vi "Begin.vi"(11 "Image Size":T1=enum."160x120") -> (0 "error out":errorcluster)   [LabVIEW 2012]
doc: "Called before other user functions, this VI is expected to open initial I/O refnums, load in file data, and do all program initialization. Notice that the <B>error out</B> terminal is simply used for data flow. Wiring it to other structures or subVIs ensures that this VI runs first."
uses:
  <vilib>/Rock Robotics/WPI/Camera/WPI_CameraImageSize.ctl
  <vilib>/Rock Robotics/WPI/Camera/WPI_CameraWhite Balance Values.ctl
  <vilib>/Rock Robotics/WPI/Camera/WPI_CameraExposure Values.ctl
  <vilib>/Rock Robotics/WPI/Camera/WPI_CameraFrameRate.ctl
  <vilib>/Rock Robotics/WPI/DriverStation/WPI_DriverStationRobotMode2.ctl
  <vilib>/Rock Robotics/SystemInterfaces/DIO/FPGA_DIOChannel.ctl
  <vilib>/Rock Robotics/SystemInterfaces/AI/FPGA_AIGyroChannel.ctl
  <vilib>/Rock Robotics/WPI/Relay/WPI_RelayDirection.ctl
  <vilib>/Rock Robotics/SystemInterfaces/DIO/FPGA_DIORelayChannel.ctl
  <vilib>/Rock Robotics/SystemInterfaces/DIO/FPGA_DIOPWMChannel.ctl
  <vilib>/Rock Robotics/WPI/Joystick/WPI_JoystickDeviceEnum.ctl
  <vilib>/Rock Robotics/SystemInterfaces/Typedef/FPGA_TypedefDigitalModule.ctl
  <vilib>/Rock Robotics/SystemInterfaces/AI/FPGA_AIChannel.ctl
  Robot Global Data.vi
  <vilib>/Rock Robotics/WPI/MotorControl/WPI_MotorControlOpen Victor.vi
  <vilib>/Rock Robotics/WPI/MotorControl/WPI_MotorControlOpen Jaguar.vi
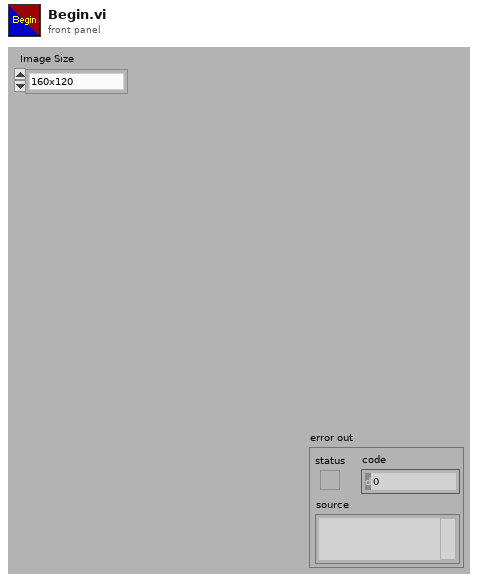
[diagram p1: front panel]
types:
  T1 = typedef "WPI_CameraImageSize.ctl" = enum16{"640x480", "320x240", "160x120"}
  T2 = typedef "FPGA_AIChannel.ctl" = enum8{"AI 1", "AI 2", "AI 3", "AI 4", "AI 5", "AI 6", "AI 7", "AI 8", "Invalid"}
  T3 = typedef "FPGA_TypedefDigitalModule.ctl" = enum16{"Digital Module 1", "Digital Module 2"}
  T4 = typedef "FPGA_DIOPWMChannel.ctl" = enum8{"PWM 1", "PWM 2", "PWM 3", "PWM 4", "PWM 5", "PWM 6", "PWM 7", "PWM 8", "PWM 9", "PWM 10", "Invalid"}
  T5 = typedef "WPI_JoystickDeviceEnum.ctl" = enum16{"USB 1", "USB 2", "USB 3", "USB 4", "Kinect 1", "Kinect 2"}
  T6 = typedef "FPGA_DIORelayChannel.ctl" = enum8{"Relay 1", "Relay 2", "Relay 3", "Relay 4", "Relay 5", "Relay 6", "Relay 7", "Relay 8", "Invalid"}
  T7 = typedef "WPI_RelayDirection.ctl" = enum16{"Both directions", "Forward only", "Reverse only"}
  T8 = typedef "FPGA_AIGyroChannel.ctl" = enum8{"AI 1", "AI 2", "Invalid"}
  T9 = typedef "FPGA_DIOChannel.ctl" = enum8{"DIO 1", "DIO 2", "DIO 3", "DIO 4", "DIO 5", "DIO 6", "DIO 7", "DIO 8", "DIO 9", "DIO 10", "DIO 11", "DIO 12", "DIO 13", "DIO 14", "Invalid"}
  T10 = typedef "WPI_DriverStationRobotMode2.ctl" = enum16{"Autonomous Disabled", "Autonomous Enabled", "Teleop Disabled", "Teleop Enabled", "Timeout", "Finish", "Test Disabled", "Test Enabled"}
  T11 = typedef "WPI_CameraFrameRate.ctl" = u32
  T12 = typedef "WPI_CameraExposure Values.ctl" = enum16{"Auto", "Flicker-free 50 Hz", "Flicker-free 60 Hz", "Hold current"}
  T13 = typedef "WPI_CameraWhite Balance Values.ctl" = enum16{"Auto", "Fixed indoor", "Fixed outdoor 1", "Fixed outdoor 2", "Fixed fluorescent 1", "Fixed fluorescent 2", "Hold current"}
  T14 = typedef "WPI_ServoDeviceRef.ctl" = cluster{"DeviceStatus":errorcluster, "Digital Module":T3, "PWM Channel":T4, "DeadBand":T15}
  T15 = typedef "WPI_PWMDeadband.ctl" = cluster{"Name":string, "maxPositivePwm":i32, "minPositivePwm":i32, "centerPwm":i32, "maxNegativePwm":i32, "minNegativePwm":i32, "angularRange":u16}
  T16 = typedef "WPI_CameraDevRef.ctl" = cluster{"Camera Address":string, "CameraStatus":errorcluster, "Acquire Image Notifier":refnum<notifier>}
  T17 = typedef "WPI_MotorControlDeviceRef.ctl" = cluster{"DeviceStatus":errorcluster, "Type":enum16{"PWM", "CAN"}, "PWM":cluster{"Digital Module":T3, "PWM Channel":T4, "DeadBand":T15}, "CAN":cluster{"Device Number":u8, "Control Mode":T18, "Semaphore":T19, "Max Vout":dbl}, "Invert":bool, "TransformRef":T20, "InvTransformRef":T20}
  T18 = typedef "WPI_CANJaguar_ControlMode.ctl" = enum8{"Percent VBus", "Current", "Speed", "Position", "Voltage"}
  T19 = typedef "Semaphore RefNum" = refnum<k1>
  T20 = typedef "WPI_PWMTransform_ConPane.ctl" = refnum<vi>
  T21 = typedef "WPI_JoystickDevRef.ctl" = cluster{"Device":T5}
  T22 = typedef "WPI_AnalogChannelDevRef.ctl" = cluster{"DevStatus":errorcluster, "Analog Module":T23, "Analog Channel":T2}
  T23 = typedef "FPGA_TypedefAnalogModule.ctl" = enum16{"Analog Module 1", "Analog Module 2"}
  T24 = typedef "WPI_RelayDevRef.ctl" = cluster{"DevStatus":errorcluster, "Relay Channel":T6, "Digital Module":T3, "Relay Direction":T7}
  T25 = typedef "WPI_DigitalInputDevRef.ctl" = cluster{"DevStatus":errorcluster, "DIO Channel":T9, "Digital Module":T3}
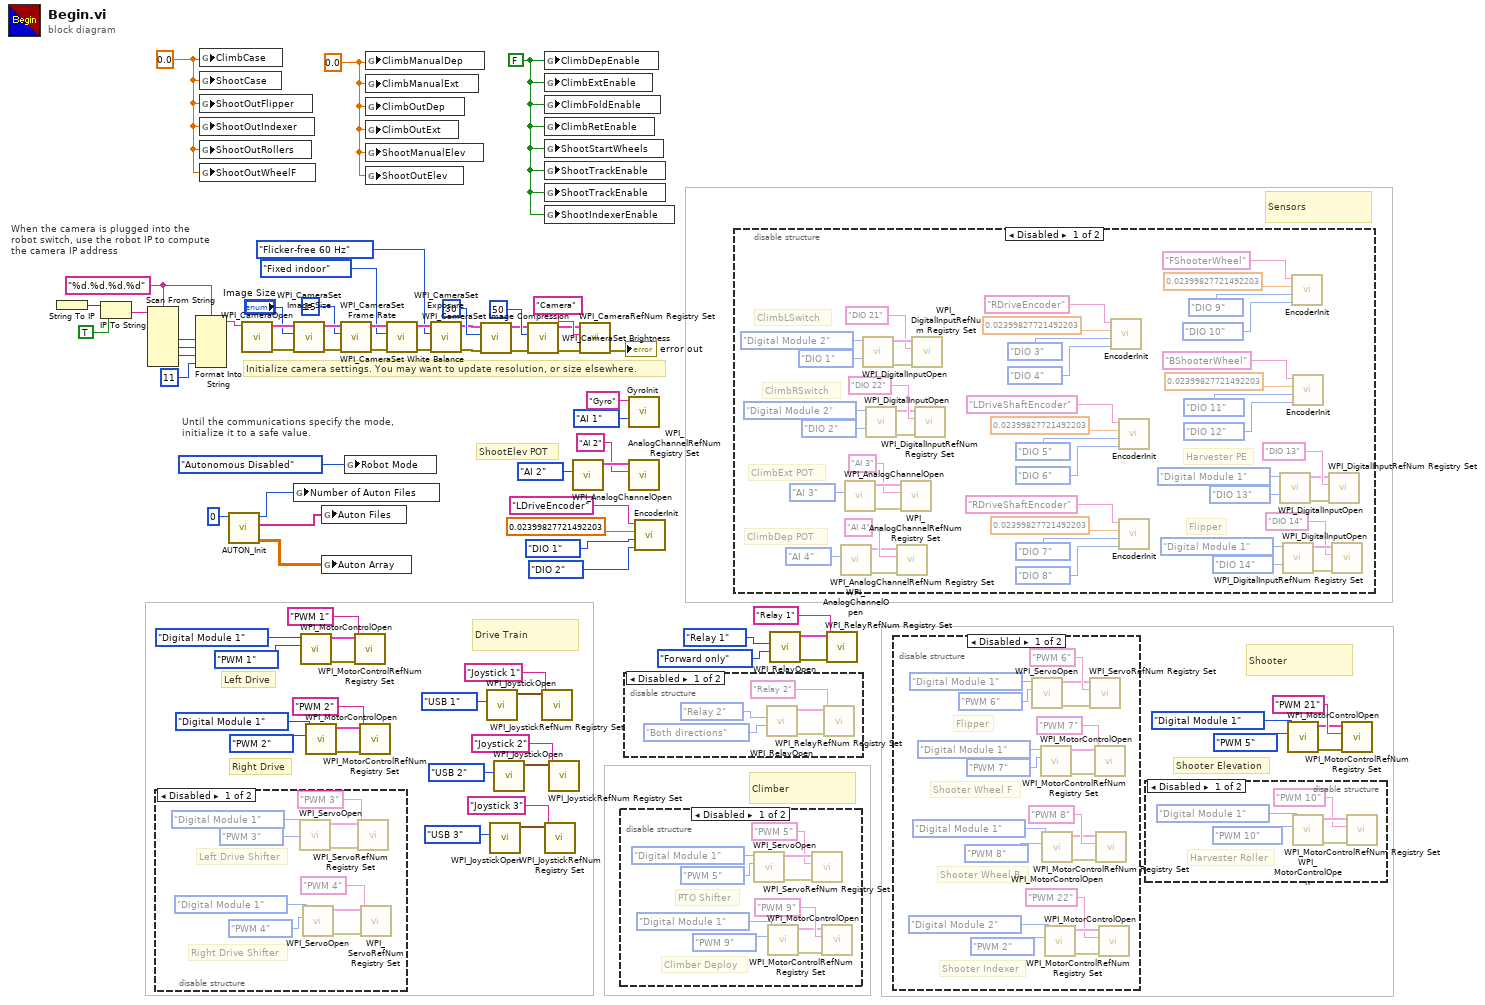
[diagram p0: block diagram]
diagram:
  w1 = FALSE ("ClimbDepEnable")
  w2 = 0.0 ("ClimbCase")
  w3 = 0.0 ("ClimbCase")
  w49 = "%d.%d.%d.%d" ("format string")
  # "ShootElev POT"
  # "Drive Train"
  # "Climber"
  # "Shooter"
  # "Shooter Elevation"
  # "Sensors"
  # "Right Drive"
  # "Left Drive"
  # "Until the communications specify the mode,\ninitialize it to a safe value."
  # "When the camera is plugged into the\nrobot switch, use the robot IP to compute\nthe camera IP address"
  # "Initialize camera settings. You may want to update resolution, or size elsewhere."
  n1 = String To IP() -> (0:w56:u32)  [unwired: 1 in]
  n2 = IP To String(1:TRUE ("dot notation? (F)"), 2:w56) -> (0:w54:string)
  n3 = Scan From String(format string=w49, input string=w54) -> (output 1=w53:i32, output 2=w52:i32, output 3=w51:i32)  [unwired: 7 in, 3 out]
  n4 = disable-structure shown="Disabled" {
    frame Disabled {
      # "Right Drive Shifter"
      # "Left Drive Shifter"
      n5 = call <vilib>:"WPI_ServoOpen.vi"("PWM Channel"=FPGA_DIOPWMChannel."PWM 3", "Digital Module (Module 1)"=FPGA_TypedefDigitalModule."Digital Module 1") -> ("error out"=w79:errorcluster, "ServoDeviceRef"=w80:T14)  [unwired: 8 in]
      n6 = call <vilib>:"WPI_ServoOpen.vi"("PWM Channel"=FPGA_DIOPWMChannel."PWM 4", "Digital Module (Module 1)"=FPGA_TypedefDigitalModule."Digital Module 1") -> ("error out"=w78:errorcluster, "ServoDeviceRef"=w85:T14)  [unwired: 8 in]
      n7 = call <vilib>:"WPI_ServoRefNum Registry Set.vi"("error in (no error)"=w79, "refnum name"="PWM 3", "ServoDeviceRef"=w80) -> ()  [unwired: 7 in, 2 out]
      n8 = call <vilib>:"WPI_ServoRefNum Registry Set.vi"("error in (no error)"=w78, "refnum name"="PWM 4", "ServoDeviceRef"=w85) -> ()  [unwired: 7 in, 2 out]
    }
    frame Enabled {
    }
  }
  n9 = Format Into String(format string=w49, w53, w52, w51, 11 ("Compression")) -> (resulting string=w47:string)  [unwired: 2 in, 1 out]
  n10 = global write "Robot Global Data.vi" "ClimbCase"(w3) -> ()
  n11 = global write "Robot Global Data.vi" "ShootCase"(w3) -> ()
  n12 = global write "Robot Global Data.vi" "ShootOutFlipper"(w3) -> ()
  n13 = global write "Robot Global Data.vi" "ShootOutIndexer"(w3) -> ()
  n14 = global write "Robot Global Data.vi" "ShootOutRollers"(w3) -> ()
  n15 = global write "Robot Global Data.vi" "ShootOutWheelF"(w3) -> ()
  n16 = call "AUTON_Init.vi"("Default File"=0) -> ("Auton Array"=w42:dbl[][], "Auton Files"=w43:string[], "Number of Auton Files"=w44:i64)  [unwired: 8 in]
  n17 = call <vilib>:"WPI_CameraOpen.vi"("Camera Address"=w47) -> ("error out"=w68:errorcluster, "CameraDevRef"=w69:T16)  [unwired: 1 in, 8 out]
  n18 = call <vilib>:"WPI_CameraSet Image Size.vi"("error in (no error)"=w68, "Image Size"="Image Size", "CameraDevRef"=w69) -> ("error out"=w67:errorcluster, "CameraDevRef Out"=w70:T16)  [unwired: 7 out]
  n19 = global write "Robot Global Data.vi" "Number of Auton Files"(w44) -> ()
  n20 = call-poly <vilib>:"WPI_MotorControlOpen.vi"("PWM Channel"=FPGA_DIOPWMChannel."PWM 1", "Digital Module (Module 1)"=FPGA_TypedefDigitalModule."Digital Module 1") -> ("error out"=w21:errorcluster, "MotorControlDeviceRef"=w22:T17)  [unwired: 8 in]
  n21 = call-poly <vilib>:"WPI_MotorControlOpen.vi"("PWM Channel"=FPGA_DIOPWMChannel."PWM 2", "Digital Module (Module 1)"=FPGA_TypedefDigitalModule."Digital Module 1") -> ("error out"=w28:errorcluster, "MotorControlDeviceRef"=w27:T17)  [unwired: 8 in]
  n22 = global write "Robot Global Data.vi" "Auton Files"(w43) -> ()
  n23 = global write "Robot Global Data.vi" "Auton Array"(w42) -> ()
  n24 = call <vilib>:"WPI_CameraSet Frame Rate.vi"("error in (no error)"=w67, "Frame Rate (fps)"=T11 15, "CameraDevRef"=w70) -> ("error out"=w66:errorcluster, "CameraDevRef Out"=w72:T16)  [unwired: 7 out]
  n25 = global write "Robot Global Data.vi" "Robot Mode"(WPI_DriverStationRobotMode2."Autonomous Disabled" ("Robot Mode")) -> ()
  n26 = call <vilib>:"WPI_MotorControlRefNum Registry Set.vi"("error in (no error)"=w21, "refnum name"="PWM 1", "MotorControlDevRef"=w22) -> ()  [unwired: 7 in, 2 out]
  n27 = call <vilib>:"WPI_MotorControlRefNum Registry Set.vi"("error in (no error)"=w28, "refnum name"="PWM 2", "MotorControlDevRef"=w27) -> ()  [unwired: 7 in, 2 out]
  n28 = global write "Robot Global Data.vi" "ClimbManualDep"(w2) -> ()
  n29 = global write "Robot Global Data.vi" "ClimbManualExt"(w2) -> ()
  n30 = global write "Robot Global Data.vi" "ClimbOutDep"(w2) -> ()
  n31 = global write "Robot Global Data.vi" "ClimbOutExt"(w2) -> ()
  n32 = global write "Robot Global Data.vi" "ShootManualElev"(w2) -> ()
  n33 = global write "Robot Global Data.vi" "ShootOutElev"(w2) -> ()
  n34 = call <vilib>:"WPI_CameraSet White Balance.vi"("error in (no error)"=w66, "White Balance"=WPI_CameraWhite_Balance_Values."Fixed indoor", "CameraDevRef"=w72) -> ("error out"=w65:errorcluster, "CameraDevRef Out"=w71:T16)  [unwired: 7 out]
  n35 = call <vilib>:"WPI_CameraSet Exposure.vi"("error in (no error)"=w65, "Exposure"=WPI_CameraExposure_Values."Flicker-free 60 Hz", "CameraDevRef"=w71) -> ("error out"=w64:errorcluster, "CameraDevRef Out"=w74:T16)  [unwired: 7 out]
  n36 = call <vilib>:"WPI_CameraSet Image Compression.vi"("error in (no error)"=w64, "Compression"=30, "CameraDevRef"=w74) -> ("error out"=w63:errorcluster, "CameraDevRef Out"=w73:T16)  [unwired: 7 out]
  n37 = call <vilib>:"WPI_JoystickOpen.vi"("JoystickDevice"=WPI_JoystickDeviceEnum."USB 1") -> ("JoystickDevRef"=w12:T21)  [unwired: 10 in]
  n38 = call <vilib>:"WPI_JoystickOpen.vi"("JoystickDevice"=WPI_JoystickDeviceEnum."USB 3") -> ("JoystickDevRef"=w18:T21)  [unwired: 10 in]
  n39 = call <vilib>:"WPI_JoystickOpen.vi"("JoystickDevice"=WPI_JoystickDeviceEnum."USB 2") -> ("JoystickDevRef"=w17:T21)  [unwired: 10 in]
  n40 = call <vilib>:"WPI_CameraSet Brightness.vi"("error in (no error)"=w63, "Brightness"=50, "CameraDevRef"=w73) -> ("error out"=w61:errorcluster, "CameraDevRef Out"=w62:T16)  [unwired: 7 out]
  n41 = call <vilib>:"WPI_JoystickRefNum Registry Set.vi"("refnum name"="Joystick 1", "JoystickDevRef"=w12) -> ()  [unwired: 8 in, 2 out]
  n42 = global write "Robot Global Data.vi" "ClimbDepEnable"(w1) -> ()
  n43 = global write "Robot Global Data.vi" "ClimbExtEnable"(w1) -> ()
  n44 = global write "Robot Global Data.vi" "ClimbFoldEnable"(w1) -> ()
  n45 = global write "Robot Global Data.vi" "ClimbRetEnable"(w1) -> ()
  n46 = global write "Robot Global Data.vi" "ShootStartWheels"(w1) -> ()
  n47 = global write "Robot Global Data.vi" "ShootTrackEnable"(w1) -> ()
  n48 = global write "Robot Global Data.vi" "ShootTrackEnable"(w1) -> ()
  n49 = global write "Robot Global Data.vi" "ShootIndexerEnable"(w1) -> ()
  n50 = call <vilib>:"WPI_JoystickRefNum Registry Set.vi"("refnum name"="Joystick 3", "JoystickDevRef"=w18) -> ()  [unwired: 8 in, 2 out]
  n51 = call <vilib>:"WPI_JoystickRefNum Registry Set.vi"("refnum name"="Joystick 2", "JoystickDevRef"=w17) -> ()  [unwired: 8 in, 2 out]
  n52 = call <vilib>:"WPI_AnalogChannelOpen.vi"("Analog Channel"=FPGA_AIChannel."AI 2") -> ("AIDeviceRef"=w6:T22)  [unwired: 9 in, 1 out]
  n53 = call <vilib>:"WPI_CameraRefNum Registry Set.vi"("error in (no error)"=w61, "refnum name"="Camera", "CameraDevRef"=w62) -> ("error out"=→"error out":errorcluster)  [unwired: 8 out]
  n54 = disable-structure shown="Disabled" {
    frame Disabled {
      # "Climber Deploy"
      # "PTO Shifter"
      n55 = call <vilib>:"WPI_ServoOpen.vi"("PWM Channel"=FPGA_DIOPWMChannel."PWM 5", "Digital Module (Module 1)"=FPGA_TypedefDigitalModule."Digital Module 1") -> ("error out"=w97:errorcluster, "ServoDeviceRef"=w96:T14)  [unwired: 8 in]
      n56 = call-poly <vilib>:"WPI_MotorControlOpen.vi"("PWM Channel"=FPGA_DIOPWMChannel."PWM 9", "Digital Module (Module 1)"=FPGA_TypedefDigitalModule."Digital Module 1") -> ("error out"=w91:errorcluster, "MotorControlDeviceRef"=w90:T17)  [unwired: 8 in]
      n57 = call <vilib>:"WPI_ServoRefNum Registry Set.vi"("error in (no error)"=w97, "refnum name"="PWM 5", "ServoDeviceRef"=w96) -> ()  [unwired: 7 in, 2 out]
      n58 = call <vilib>:"WPI_MotorControlRefNum Registry Set.vi"("error in (no error)"=w91, "refnum name"="PWM 9", "MotorControlDevRef"=w90) -> ()  [unwired: 7 in, 2 out]
    }
    frame Enabled {
    }
  }
  n59 = disable-structure shown="Disabled" {
    frame Disabled {
      n60 = call <vilib>:"WPI_RelayOpen.vi"("Relay Direction"=WPI_RelayDirection."Both directions", "Relay Channel"=FPGA_DIORelayChannel."Relay 2") -> ("error out"=w98:errorcluster, "RelayDevRef"=w99:T24)  [unwired: 8 in]
      n61 = call <vilib>:"WPI_RelayRefNum Registry Set.vi"("error in (no error)"=w98, "refnum name"="Relay 2", "RelayDevRef"=w99) -> ()  [unwired: 7 in, 2 out]
    }
    frame Enabled {
    }
  }
  n62 = call "GyroInit.vi"("refnum name"="Gyro", "Analog Channel"=FPGA_AIGyroChannel."AI 1") -> ()  [unwired: 8 in]
  n63 = call <vilib>:"WPI_AnalogChannelRefNum Registry Set.vi"("refnum name"="AI 2", "AIDeviceRef"=w6) -> ()  [unwired: 8 in, 2 out]
  n64 = call "EncoderInit.vi"("refnum name"="LDriveEncoder", "DistancePerCount"=0.02399827721492203, "DIO Channel"=FPGA_DIOChannel."DIO 1", "DIO Channel 2"=FPGA_DIOChannel."DIO 2") -> ()  [unwired: 7 in]
  n65 = disable-structure shown="Disabled" {
    frame Disabled {
      # "ClimbRSwitch"
      # "ClimbLSwitch"
      # "ClimbDep POT"
      # "ClimbExt POT"
      # "Flipper"
      # "Harvester PE"
      n66 = call <vilib>:"WPI_AnalogChannelOpen.vi"("Analog Channel"=FPGA_AIChannel."AI 4") -> ("error out"=w117:errorcluster, "AIDeviceRef"=w118:T22)  [unwired: 9 in]
      n67 = call <vilib>:"WPI_AnalogChannelOpen.vi"("Analog Channel"=FPGA_AIChannel."AI 3") -> ("error out"=w116:errorcluster, "AIDeviceRef"=w115:T22)  [unwired: 9 in]
      n68 = call <vilib>:"WPI_DigitalInputOpen.vi"("DIO Channel"=FPGA_DIOChannel."DIO 1", "Digital Module (Module 1)"=FPGA_TypedefDigitalModule."Digital Module 2") -> ("error out"=w104:errorcluster, "DigitalInputDevRef"=w105:T25)  [unwired: 8 in]
      n69 = call <vilib>:"WPI_DigitalInputOpen.vi"("DIO Channel"=FPGA_DIOChannel."DIO 2", "Digital Module (Module 1)"=FPGA_TypedefDigitalModule."Digital Module 2") -> ("error out"=w111:errorcluster, "DigitalInputDevRef"=w110:T25)  [unwired: 8 in]
      n70 = call <vilib>:"WPI_AnalogChannelRefNum Registry Set.vi"("error in (no error)"=w117, "refnum name"="AI 4", "AIDeviceRef"=w118) -> ()  [unwired: 7 in, 2 out]
      n71 = call <vilib>:"WPI_AnalogChannelRefNum Registry Set.vi"("error in (no error)"=w116, "refnum name"="AI 3", "AIDeviceRef"=w115) -> ()  [unwired: 7 in, 2 out]
      n72 = call <vilib>:"WPI_DigitalInputRefNum Registry Set.vi"("error in (no error)"=w104, "refnum name"="DIO 21", "DigitalInputDevRef"=w105) -> ()  [unwired: 7 in, 2 out]
      n73 = call <vilib>:"WPI_DigitalInputRefNum Registry Set.vi"("error in (no error)"=w111, "refnum name"="DIO 22", "DigitalInputDevRef"=w110) -> ()  [unwired: 7 in, 2 out]
      n74 = call "EncoderInit.vi"("refnum name"="RDriveEncoder", "DistancePerCount"=0.02399827721492203, "DIO Channel"=FPGA_DIOChannel."DIO 3", "DIO Channel 2"=FPGA_DIOChannel."DIO 4") -> ()  [unwired: 7 in]
      n75 = call "EncoderInit.vi"("refnum name"="LDriveShaftEncoder", "DistancePerCount"=0.02399827721492203, "DIO Channel"=FPGA_DIOChannel."DIO 5", "DIO Channel 2"=FPGA_DIOChannel."DIO 6") -> ()  [unwired: 7 in]
      n76 = call "EncoderInit.vi"("refnum name"="RDriveShaftEncoder", "DistancePerCount"=0.02399827721492203, "DIO Channel"=FPGA_DIOChannel."DIO 7", "DIO Channel 2"=FPGA_DIOChannel."DIO 8") -> ()  [unwired: 7 in]
      n77 = call <vilib>:"WPI_DigitalInputOpen.vi"("DIO Channel"=FPGA_DIOChannel."DIO 13", "Digital Module (Module 1)"=FPGA_TypedefDigitalModule."Digital Module 1") -> ("error out"=w129:errorcluster, "DigitalInputDevRef"=w128:T25)  [unwired: 8 in]
      n78 = call <vilib>:"WPI_DigitalInputOpen.vi"("DIO Channel"=FPGA_DIOChannel."DIO 14", "Digital Module (Module 1)"=FPGA_TypedefDigitalModule."Digital Module 1") -> ("error out"=w122:errorcluster, "DigitalInputDevRef"=w123:T25)  [unwired: 8 in]
      n79 = call "EncoderInit.vi"("refnum name"="FShooterWheel", "DistancePerCount"=0.02399827721492203, "DIO Channel"=FPGA_DIOChannel."DIO 9", "DIO Channel 2"=FPGA_DIOChannel."DIO 10") -> ()  [unwired: 7 in]
      n80 = call "EncoderInit.vi"("refnum name"="BShooterWheel", "DistancePerCount"=0.02399827721492203, "DIO Channel"=FPGA_DIOChannel."DIO 11", "DIO Channel 2"=FPGA_DIOChannel."DIO 12") -> ()  [unwired: 7 in]
      n81 = call <vilib>:"WPI_DigitalInputRefNum Registry Set.vi"("error in (no error)"=w129, "refnum name"="DIO 13", "DigitalInputDevRef"=w128) -> ()  [unwired: 7 in, 2 out]
      n82 = call <vilib>:"WPI_DigitalInputRefNum Registry Set.vi"("error in (no error)"=w122, "refnum name"="DIO 14", "DigitalInputDevRef"=w123) -> ()  [unwired: 7 in, 2 out]
    }
    frame Enabled {
    }
  }
  n83 = call <vilib>:"WPI_RelayOpen.vi"("Relay Direction"=WPI_RelayDirection."Forward only", "Relay Channel"=FPGA_DIORelayChannel."Relay 1") -> ("error out"=w35:errorcluster, "RelayDevRef"=w34:T24)  [unwired: 8 in]
  n84 = call <vilib>:"WPI_RelayRefNum Registry Set.vi"("error in (no error)"=w35, "refnum name"="Relay 1", "RelayDevRef"=w34) -> ()  [unwired: 7 in, 2 out]
  n85 = disable-structure shown="Disabled" {
    frame Disabled {
      # "Shooter Wheel B"
      # "Flipper"
      # "Shooter Indexer"
      # "Shooter Wheel F"
      n86 = call <vilib>:"WPI_ServoOpen.vi"("PWM Channel"=FPGA_DIOPWMChannel."PWM 6", "Digital Module (Module 1)"=FPGA_TypedefDigitalModule."Digital Module 1") -> ("error out"=w156:errorcluster, "ServoDeviceRef"=w157:T14)  [unwired: 8 in]
      n87 = call-poly <vilib>:"WPI_MotorControlOpen.vi"("PWM Channel"=FPGA_DIOPWMChannel."PWM 7", "Digital Module (Module 1)"=FPGA_TypedefDigitalModule."Digital Module 1") -> ("error out"=w167:errorcluster, "MotorControlDeviceRef"=w168:T17)  [unwired: 8 in]
      n88 = call-poly <vilib>:"WPI_MotorControlOpen.vi"("PWM Channel"=FPGA_DIOPWMChannel."PWM 8", "Digital Module (Module 1)"=FPGA_TypedefDigitalModule."Digital Module 1") -> ("error out"=w153:errorcluster, "MotorControlDeviceRef"=w152:T17)  [unwired: 8 in]
      n89 = call-poly <vilib>:"WPI_MotorControlOpen.vi"("PWM Channel"=FPGA_DIOPWMChannel."PWM 2", "Digital Module (Module 1)"=FPGA_TypedefDigitalModule."Digital Module 2") -> ("error out"=w163:errorcluster, "MotorControlDeviceRef"=w164:T17)  [unwired: 8 in]
      n90 = call <vilib>:"WPI_ServoRefNum Registry Set.vi"("error in (no error)"=w156, "refnum name"="PWM 6", "ServoDeviceRef"=w157) -> ()  [unwired: 7 in, 2 out]
      n91 = call <vilib>:"WPI_MotorControlRefNum Registry Set.vi"("error in (no error)"=w167, "refnum name"="PWM 7", "MotorControlDevRef"=w168) -> ()  [unwired: 7 in, 2 out]
      n92 = call <vilib>:"WPI_MotorControlRefNum Registry Set.vi"("error in (no error)"=w153, "refnum name"="PWM 8", "MotorControlDevRef"=w152) -> ()  [unwired: 7 in, 2 out]
      n93 = call <vilib>:"WPI_MotorControlRefNum Registry Set.vi"("error in (no error)"=w163, "refnum name"="PWM 22", "MotorControlDevRef"=w164) -> ()  [unwired: 7 in, 2 out]
    }
    frame Enabled {
    }
  }
  n94 = disable-structure shown="Disabled" {
    frame Disabled {
      # "Harvester Roller"
      n95 = call-poly <vilib>:"WPI_MotorControlOpen.vi"("PWM Channel"=FPGA_DIOPWMChannel."PWM 10", "Digital Module (Module 1)"=FPGA_TypedefDigitalModule."Digital Module 1") -> ("error out"=w173:errorcluster, "MotorControlDeviceRef"=w174:T17)  [unwired: 8 in]
      n96 = call <vilib>:"WPI_MotorControlRefNum Registry Set.vi"("error in (no error)"=w173, "refnum name"="PWM 10", "MotorControlDevRef"=w174) -> ()  [unwired: 7 in, 2 out]
    }
    frame Enabled {
    }
  }
  n97 = call-poly <vilib>:"WPI_MotorControlOpen.vi"("PWM Channel"=FPGA_DIOPWMChannel."PWM 5", "Digital Module (Module 1)"=FPGA_TypedefDigitalModule."Digital Module 1") -> ("error out"=w9:errorcluster, "MotorControlDeviceRef"=w8:T17)  [unwired: 8 in]
  n98 = call <vilib>:"WPI_MotorControlRefNum Registry Set.vi"("error in (no error)"=w9, "refnum name"="PWM 21", "MotorControlDevRef"=w8) -> ()  [unwired: 7 in, 2 out]
